vi "Process.vi"(8 "error in (no error)":errorcluster, 10 "Stop Msg in":refnum<class "Stop Msg.lvclass">, 11 "Architecture.lvlib:Thread.lvclass":refnum<class "Thread.lvclass">) -> (0 "error out":errorcluster, 1 "Stop?":bool, 3 "Architecture.lvlib:Thread.lvclass 2":refnum<class "Thread.lvclass">)   [LabVIEW 2016, in "Architecture.lvlib" / "Stop Msg.lvclass"]
uses:
  Stop Msg.lvclass
  Thread/Thread.lvclass
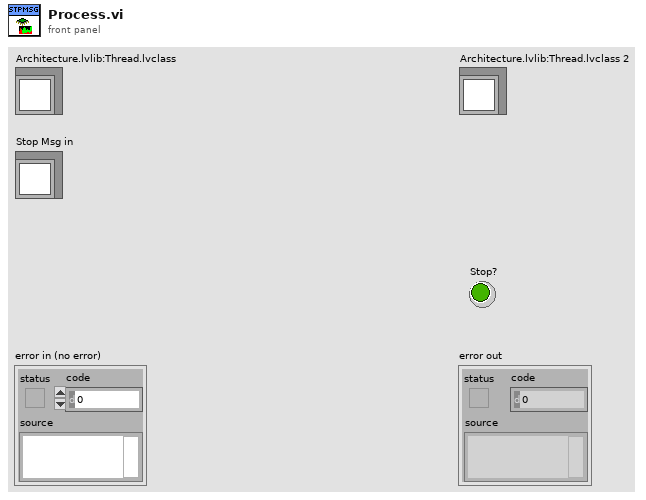
[diagram p1: front panel]
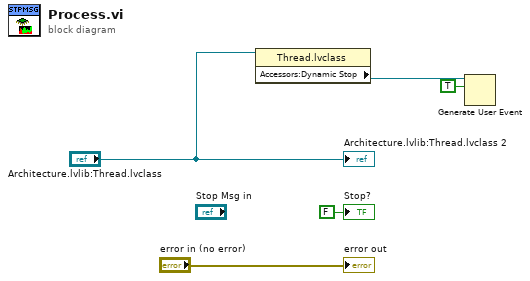
[diagram p0: block diagram]
diagram:
  n1 = property class="Thread.lvclass"(reference="Architecture.lvlib:Thread.lvclass") -> ("Accessors:Dynamic Stop"=w2:refnum<user-event>)  [unwired: 1 in, 2 out]
  n2 = Generate User Event(user event=w2, event data cluster=TRUE ("event data")) -> ()  [unwired: 2 in, 2 out]
  "error out" <- "error in (no error)"
  "Stop?" <- FALSE ("Stop?")
  "Architecture.lvlib:Thread.lvclass 2" <- "Architecture.lvlib:Thread.lvclass"
